vi "ReadSectionCacheData.vi"(8 "error in (no error)":errorcluster, 9 "section":string, 11 "Refnum in":T1) -> (0 "error out":errorcluster, 2 "CacheRecreateDuration":dbl, 3 "refnum out":T1)   [LabVIEW 2019, in "Hawkeye.lvlib"]
uses:
  Hawkeye.lvlib
  <vilib>/Utility/config.llb/Config Data RefNum.ctl
  <vilib>/Utility/config.llb/Read Key (Double).vi
  <vilib>/Utility/config.llb/NI_LVConfig.lvlib
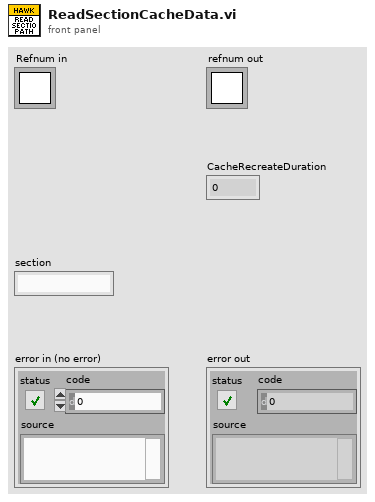
[diagram p1: front panel]
types:
  T1 = typedef "NI_LVConfig.lvlib/Config Data RefNum.ctl" = refnum<k1>
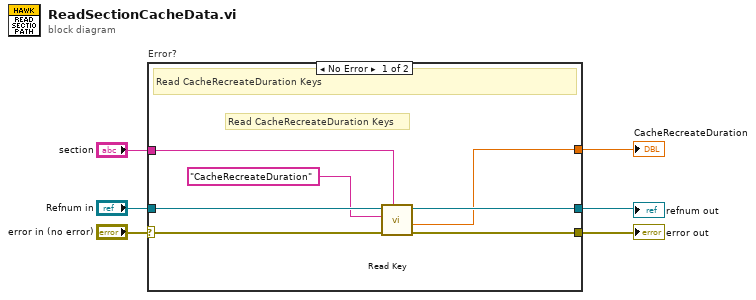
[diagram p0: block diagram]
diagram:
  n1 = case "Error?" shown="No Error" "error in (no error)" {
    selector: "error in (no error)" -> [w12 w14]
    tunnel: "section" -> [w13 _]
    tunnel: "Refnum in" -> [w11 w15]
    tunnel: [w9 w14] -> w3
    tunnel: [w8 w15] -> w2
    tunnel: [w7 _] -> w1
    frame No Error {
      # "Read CacheRecreateDuration Keys"
      # "Read CacheRecreateDuration Keys"
      n2 = call-poly <vilib>:"Read Key.vi"("section"=w13, "error in (no error)"=w12, "key"="CacheRecreateDuration", "refnum"=w11) -> ("error out"=w9:errorcluster, "value"=w7:dbl, "refnum out"=w8:T1)  [unwired: 4 in, 1 out]
    }
    frame Error {
      # "Error"
    }
  }
  "refnum out" <- w2
  "error out" <- w3
  "CacheRecreateDuration" <- w1
